vi "ReleaseStateQueue.vi"(8 "error in (no error)":errorcluster, 11 "QueueIn":variant) -> (0 "error out":errorcluster)   [LabVIEW 2013]
uses:
  SysControl/States.ctl
panel:
  in  "queue out":refnum<queue>
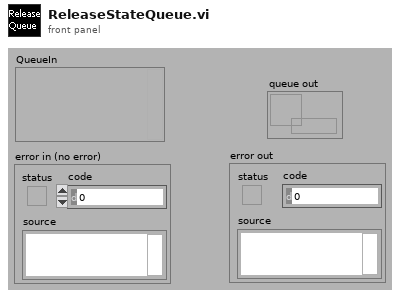
[diagram p1: front panel]
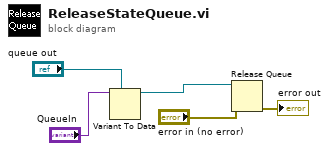
[diagram p0: block diagram]
diagram:
  n1 = Variant To Data(type="queue out", Variant="QueueIn") -> (data=w3:refnum<queue>)  [unwired: 1 in, 1 out]
  n2 = Release Queue(queue=w3, error in (no error)="error in (no error)") -> (error out=→"error out":errorcluster)  [unwired: 3 out]
